vi "Handle 44_1_2.vi"(8 "error in (no error)":errorcluster, 11 "Stand in":refnum<class "Stand.lvclass">) -> (0 "error out":errorcluster, 3 "Stand out":refnum<class "Stand.lvclass">)   [LabVIEW 2019, in "Stand.lvclass"]
uses:
  Stand.lvclass
  Stand.lvclass/Stand.ctl
  TypeDef/State 44-1-2.ctl
  Valve_2DO_2DI_class/Valve_2DO_2DI.lvclass/Valve_2DO_2DI.ctl
  Device_class/Device.lvclass/Device.ctl
  53daa488-cb92-467d-8939-09c81072894d.vi
  27880750-5bda-4793-8800-8ef0418d5d30.vi
  Device_class/GetFPGA.vi
  Valve_2DO_2DI_class/Valve_2DO_2DI.lvclass
  C:/Users/ANENKOV_V1/Desktop/src/Device_class/Device.lvclass
  FPGA_API_class/FPGA API.lvclass
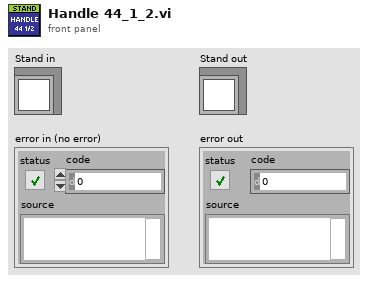
[diagram p1: front panel]
types:
  T1 = typedef "State 44-1-2.ctl" = enum16{"Init", "Idle", "Wait", "Open 44-1", "Open 44-2", "Close 44-1", "Close 44-2"}
  T2 = typedef "valveState.ctl" = enum16{"Unknown", "Closed", "Opening", "Opened", "Closing"}
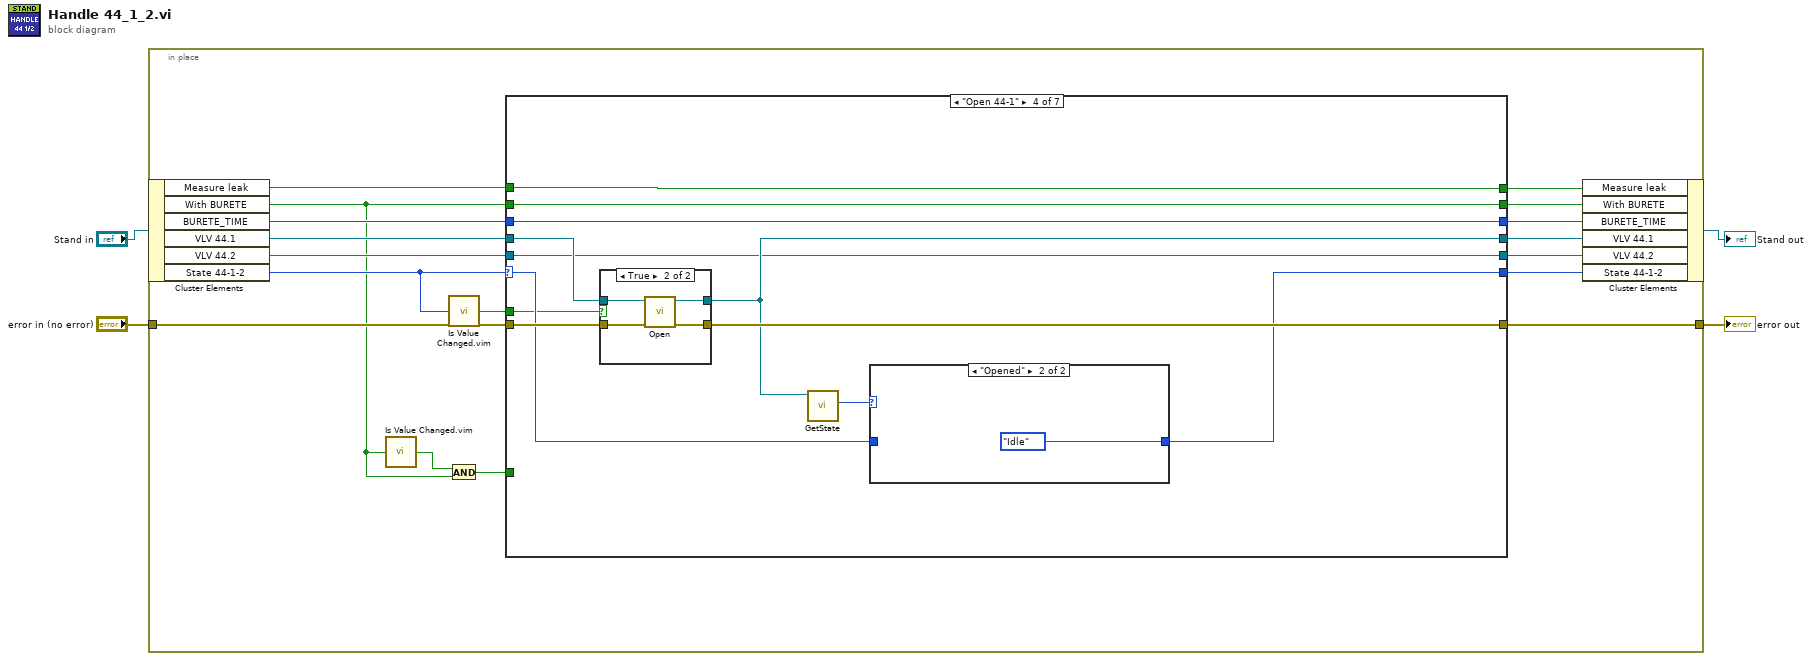
[diagram p0: block diagram]
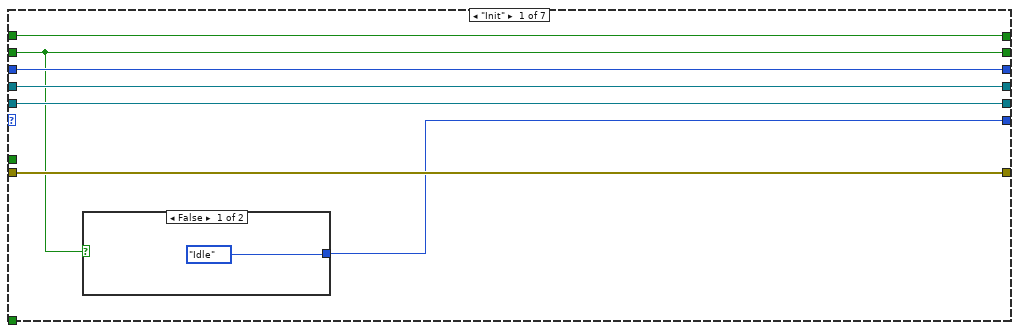
[diagram p2: hidden frame]
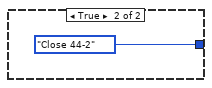
[diagram p3: hidden frame]
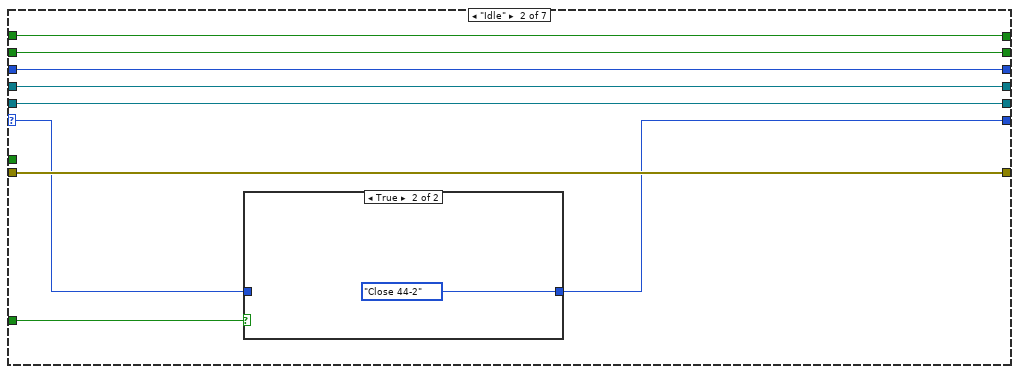
[diagram p4: hidden frame]
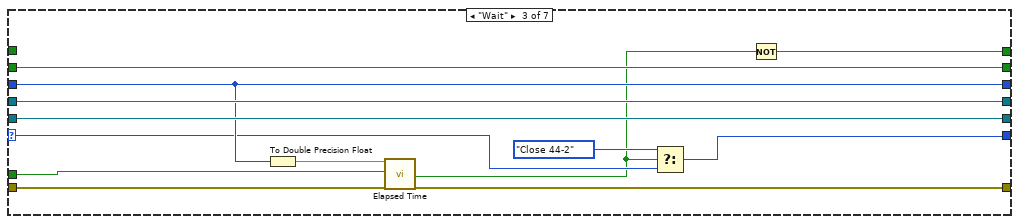
[diagram p6: hidden frame]
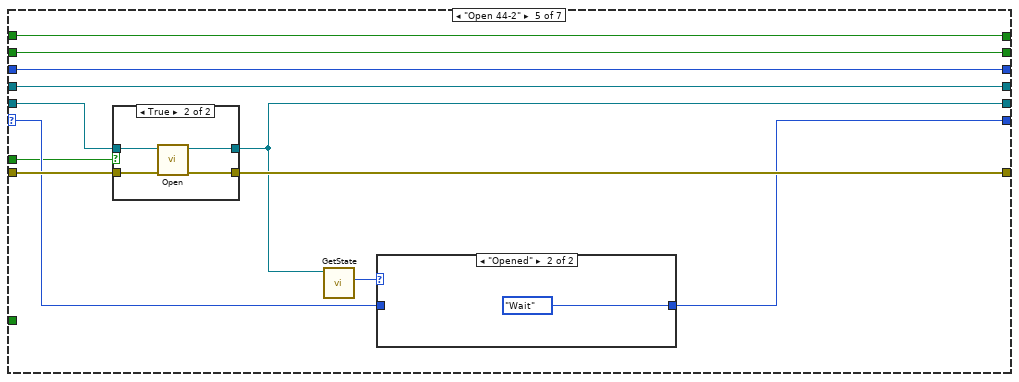
[diagram p9: hidden frame]
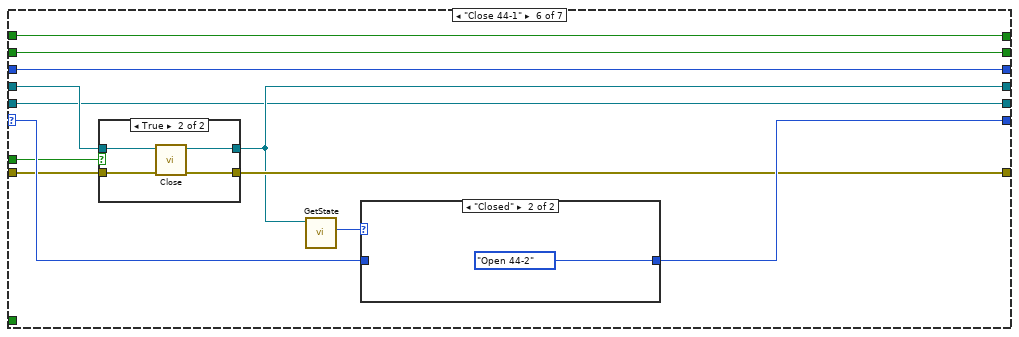
[diagram p12: hidden frame]
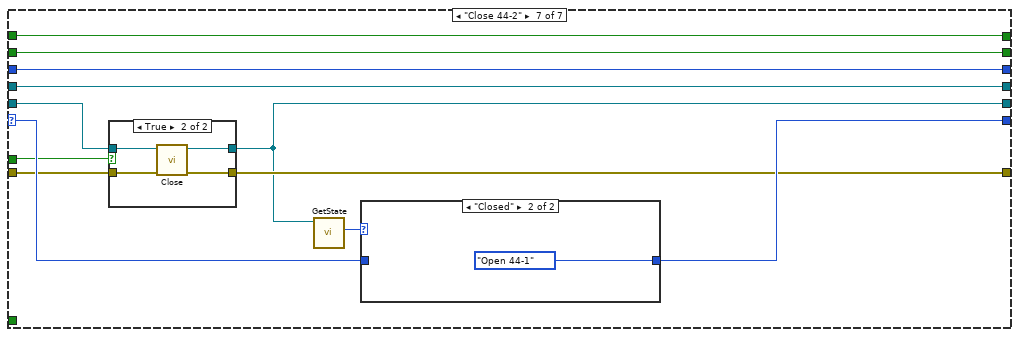
[diagram p15: hidden frame]
diagram:
  n1 = in-place {
    in-place-border: "error in (no error)" -> [w20]
    in-place-border: [w18] -> w1
    n2 = in-place-cluster #1("Stand in") -> ("Measure leak"=w5:bool, "With BURETE"=w8:bool, "BURETE_TIME"=w14:u16, "VLV 44.1"=w21:refnum<class "Valve_2DO_2DI.lvclass">, "VLV 44.2"=w16:refnum<class "Valve_2DO_2DI.lvclass">, "State 44-1-2"=w13:T1)
    n3 = call "Is Value Changed.vim"("value"=w8) -> ("changed or first call?"=w9:bool)
    n4 = call "Is Value Changed.vim"("value"=w13) -> ("changed or first call?"=w12:bool)
    n5 = And(x=w9, y=w8) -> (x .and. y?=w7:bool)
    n6 = case shown="\"Open 44-1\"" w13 {
      selector: w13 -> [_ w34 w47 w63 w83 w105 w125]
      tunnel: w21 -> [w27 w39 w54 w59 w78 w99 w119]
      tunnel: w20 -> [w25 w38 w50 w66 w86 w103 w123]
      tunnel: [w27 w39 w54 w58 w78 w98 w119] -> w19
      tunnel: [w25 w38 w48 w65 w85 w102 w122] -> w18
      tunnel: [w26 w37 w53 w57 w77 w97 w117] -> w17
      tunnel: w16 -> [w26 w37 w53 w57 w79 w97 w118]
      tunnel: [w23 w33 w45 w62 w82 w104 w124] -> w15
      tunnel: w14 -> [w28 w36 w52 w61 w81 w101 w121]
      tunnel: w12 -> [_ _ w49 w56 w76 w96 w116]
      tunnel: w8 -> [w24 w35 w44 w60 w80 w100 w120]
      tunnel: [w28 w36 w52 w61 w81 w101 w121] -> w11
      tunnel: [w24 w35 w44 w60 w80 w100 w120] -> w10
      tunnel: w7 -> [_ w32 _ _ _ _ _]
      tunnel: [w22 w31 w42 w55 w75 w95 w115] -> w6
      tunnel: w5 -> [w22 w31 _ w55 w75 w95 w115]
      frame "Init" {
        n7 = case shown="False" w24 {
          tunnel: [State_44-1-2."Idle" ("f") State_44-1-2."Close 44-2" ("State 44-1-2")] -> w23
          frame False {
          }
          frame True {
          }
        }
      }
      frame "Idle" {
        n8 = case shown="True" w32 {
          tunnel: w34 -> [w40 _]
          tunnel: [w40 State_44-1-2."Close 44-2" ("State 44-1-2")] -> w33
          frame False {
          }
          frame True {
          }
        }
      }
      frame "Wait" {
        n9 = To Double Precision Float(number=w52) -> (double precision float=w51:dbl)
        n10 = call "Elapsed Time"("Time Target (s)"=w51, "Reset"=w49, "error in (no error)"=w50) -> ("Time has Elapsed"=w43:bool, "error out"=w48:errorcluster)  [unwired: 9 in, 6 out]
        n11 = Select(t=State_44-1-2."Close 44-2", s=w43, f=w47) -> (s? t:f=w45:T1)
        n12 = Not(x=w43) -> (.not. x?=w42:bool)
      }
      frame "Open 44-1" {
        n13 = case shown="True" w56 {
          tunnel: w66 -> [w67 w72]
          tunnel: [w67 w71] -> w65
          tunnel: w59 -> [w68 w70]
          tunnel: [w68 w69] -> w58
          frame False {
          }
          frame True {
            n14 = call "Open.vi"("error in (no error)"=w72, "Pump_1AI_1DO_2DI in"=w70) -> ("error out"=w71:errorcluster, "Pump_1AI_1DO_2DI out"=w69:refnum<class "Valve_2DO_2DI.lvclass">)  [unwired: 8 in]
          }
        }
        n15 = call "GetState.vi"("Pump_1AI_1DO_2DI in"=w58) -> ("valveState"=w64:T2)  [unwired: 10 in]
        n16 = case shown="\"Opened\"" w64 {
          tunnel: w63 -> [w73 _]
          tunnel: [w73 State_44-1-2."Idle" ("State 44-1-2")] -> w62
          frame Default {
          }
          frame "Opened" {
          }
        }
      }
      frame "Open 44-2" {
        n17 = case shown="True" w76 {
          tunnel: w86 -> [w87 w92]
          tunnel: [w87 w91] -> w85
          tunnel: w79 -> [w88 w90]
          tunnel: [w88 w89] -> w77
          frame False {
          }
          frame True {
            n18 = call "Open.vi"("error in (no error)"=w92, "Pump_1AI_1DO_2DI in"=w90) -> ("error out"=w91:errorcluster, "Pump_1AI_1DO_2DI out"=w89:refnum<class "Valve_2DO_2DI.lvclass">)  [unwired: 8 in]
          }
        }
        n19 = call "GetState.vi"("Pump_1AI_1DO_2DI in"=w77) -> ("valveState"=w84:T2)  [unwired: 10 in]
        n20 = case shown="\"Opened\"" w84 {
          tunnel: w83 -> [w93 _]
          tunnel: [w93 State_44-1-2."Wait" ("State 44-1-2")] -> w82
          frame Default {
          }
          frame "Opened" {
          }
        }
      }
      frame "Close 44-1" {
        n21 = case shown="True" w96 {
          tunnel: w103 -> [w107 w112]
          tunnel: [w107 w111] -> w102
          tunnel: w99 -> [w108 w110]
          tunnel: [w108 w109] -> w98
          frame False {
          }
          frame True {
            n22 = call "Close.vi"("error in (no error)"=w112, "Pump_1AI_1DO_2DI in"=w110) -> ("error out"=w111:errorcluster, "Pump_1AI_1DO_2DI out"=w109:refnum<class "Valve_2DO_2DI.lvclass">)  [unwired: 8 in]
          }
        }
        n23 = call "GetState.vi"("Pump_1AI_1DO_2DI in"=w98) -> ("valveState"=w106:T2)  [unwired: 10 in]
        n24 = case shown="\"Closed\"" w106 {
          tunnel: w105 -> [w113 _]
          tunnel: [w113 State_44-1-2."Open 44-2" ("State 44-1-2")] -> w104
          frame Default {
          }
          frame "Closed" {
          }
        }
      }
      frame "Close 44-2" {
        n25 = case shown="True" w116 {
          tunnel: w123 -> [w127 w132]
          tunnel: [w127 w131] -> w122
          tunnel: w118 -> [w128 w130]
          tunnel: [w128 w129] -> w117
          frame False {
          }
          frame True {
            n26 = call "Close.vi"("error in (no error)"=w132, "Pump_1AI_1DO_2DI in"=w130) -> ("error out"=w131:errorcluster, "Pump_1AI_1DO_2DI out"=w129:refnum<class "Valve_2DO_2DI.lvclass">)  [unwired: 8 in]
          }
        }
        n27 = call "GetState.vi"("Pump_1AI_1DO_2DI in"=w117) -> ("valveState"=w126:T2)  [unwired: 10 in]
        n28 = case shown="\"Closed\"" w126 {
          tunnel: w125 -> [w133 _]
          tunnel: [w133 State_44-1-2."Open 44-1" ("State 44-1-2")] -> w124
          frame Default {
          }
          frame "Closed" {
          }
        }
      }
    }
    n29 = in-place-cluster #1("Measure leak"=w6, "With BURETE"=w10, "BURETE_TIME"=w11, "VLV 44.1"=w19, "VLV 44.2"=w17, "State 44-1-2"=w15) -> (→"Stand out":refnum<class "Stand.lvclass">)
  }
  "error out" <- w1
